vi "GetTreeColTxt.vi"(8 "ErrorIn(No Error)":errorcluster caption="entrée d'erreur (pas d'erreur)", 9 "Column":i32=1, 10 "CellTag":string, 11 "TreeRef":refnum<vi>) -> (0 "sortie d'erreur":errorcluster, 2 "Cellule active : chaîne":string, 3 "TreeRef":refnum<vi>)   [LabVIEW 2019]
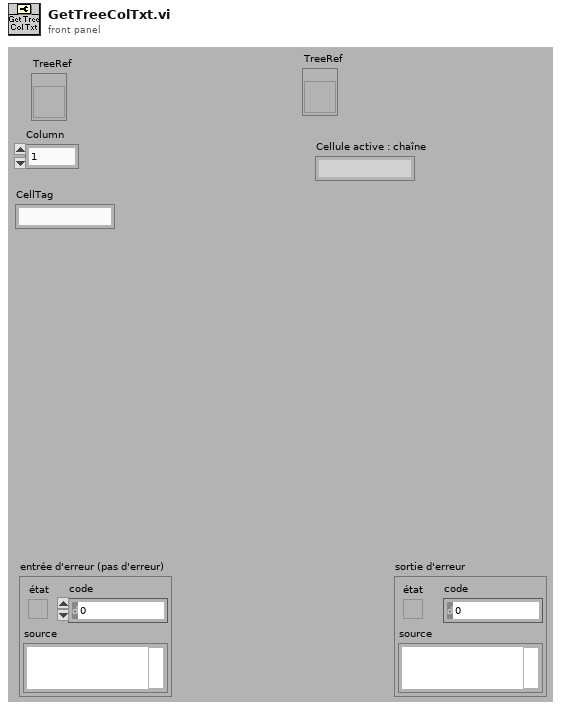
[diagram p1: front panel]
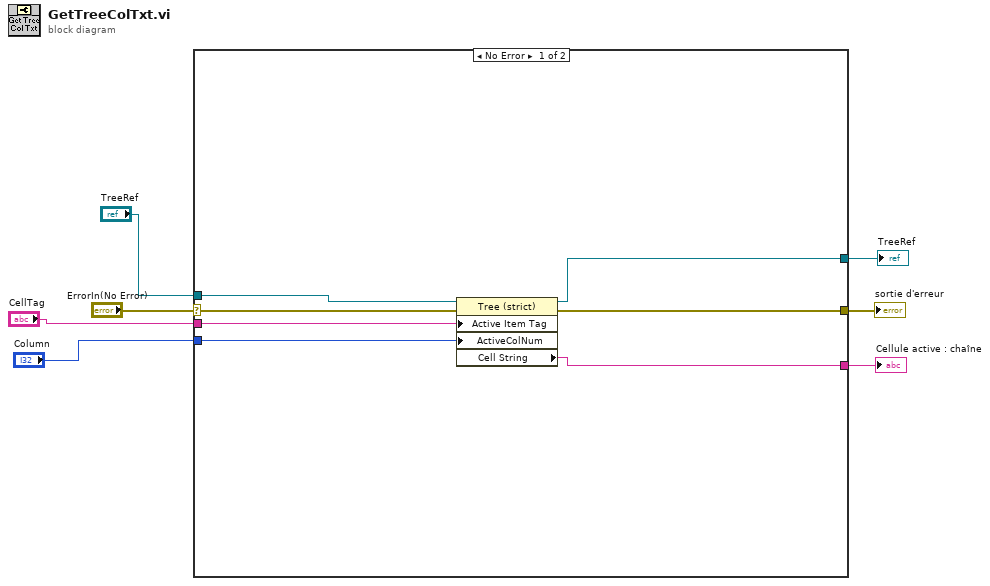
[diagram p0: block diagram]
diagram:
  n1 = case shown="No Error" "ErrorIn(No Error)" {
    selector: "ErrorIn(No Error)" -> [w14 w15]
    tunnel: [w13 w15] -> w6
    tunnel: "TreeRef" -> [w12 _]
    tunnel: "Column" -> [w11 _]
    tunnel: "CellTag" -> [w10 _]
    tunnel: [w9 _] -> w2
    tunnel: [w8 _] -> w1
    frame No Error {
      n2 = property on="Nœud de propriété" class="Tree (strict)"(reference=w12, error in=w14, "Active Item Tag"=w10, "ActiveColNum"=w11) -> (reference out=w8:refnum<vi>, error out=w13:errorcluster, "Cell String"=w9:string)
    }
    frame Error {
    }
  }
  "sortie d'erreur" <- w6
  "TreeRef" <- w1
  "Cellule active : chaîne" <- w2
